vi "Pivot Position_wrapper.vi"(11 "Pivot Position":T4) -> ()   [LabVIEW 2019]
uses:
  <vilib>/Rock Robotics/WPI/Framework/Command Status Info.ctl
  <vilib>/Rock Robotics/WPI/Framework/Completion Status.ctl
  <vilib>/Rock Robotics/WPI/Framework/Completion Notifier.ctl
  Intake Support Code/Pivot Position.ctl
panel:
  out "Command Info Out":T1
  in  "Command Info In":T1
  in  "Description":string
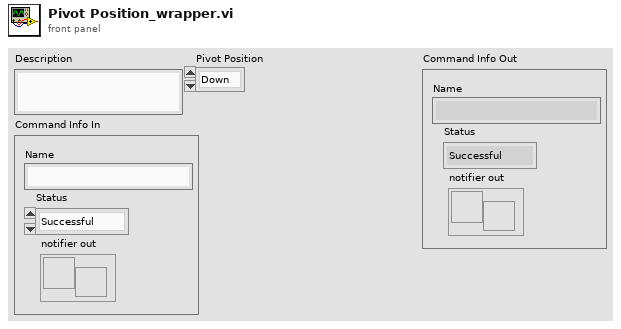
[diagram p1: front panel]
types:
  T1 = typedef "Command Status Info.ctl" = cluster{"Name":string, "Status":T2, "notifier out":T3}
  T2 = typedef "Completion Status.ctl" = enum16{"Successful", "Aborted", "Incomplete"}
  T3 = typedef "Completion Notifier.ctl" = refnum<notifier>
  T4 = typedef "Pivot Position.ctl" = enum16{"Down", "Up"}
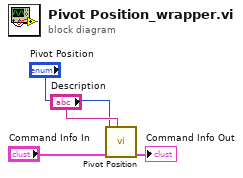
[diagram p0: block diagram]
diagram:
  n1 = call "Pivot Position.vi"("Description"="Description", "Command Info In"="Command Info In", "Pivot Position"="Pivot Position") -> ("Command Info Out"=→"Command Info Out":T1)  [unwired: 8 in]
